vi "MGCC_Commun_lowpassfilter_BESS.vi"(7 "Col":i32) -> ()   [LabVIEW 2016]
uses:
  <vilib>/Analysis/baseanly.llb/Mean (DBL).vi
  Global communication.vi
  <vilib>/Analysis/NI_AALBase.lvlib
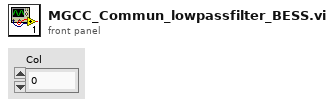
[diagram p1: front panel]
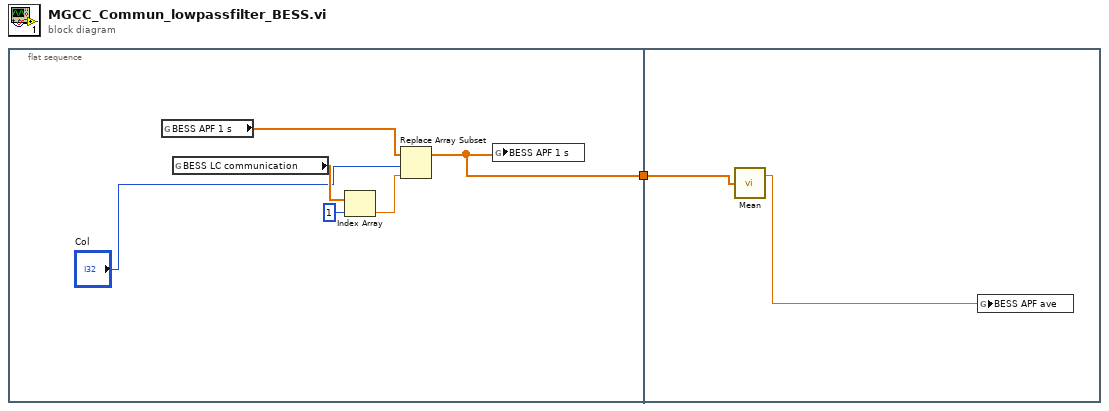
[diagram p0: block diagram]
diagram:
  n1 = flat-sequence {
    tunnel: [w6] -> w1
    tunnel: w1 -> [w9]
    frame #0 {
      n2 = global read "Global communication.vi" "BESS APF 1 s"() -> (w7:dbl[])
      n3 = global read "Global communication.vi" "BESS LC communication"() -> (w5:dbl[])
      n4 = Index Array(array=w5, index=1) -> (element=w3:dbl)
      n5 = Replace Array Subset(array=w7, new element=w3, index="Col") -> (w6:dbl[])
      n6 = global write "Global communication.vi" "BESS APF 1 s"(w6) -> ()
    }
    frame #1 {
      n7 = call-poly <vilib>:"Mean.vi"("X"=w9) -> ("mean"=w8:dbl)  [unwired: 1 out]
      n8 = global write "Global communication.vi" "BESS APF ave"(w8) -> ()
    }
  }
